vi "Redundant_Main_Micro_Comm.vi"(0 "GEA2 Reference In":refnum<k24>, 1 "GEA Inputs":T1 {"Destination" format="%.0x"; "Source" format="%.0x"}, 2 "Standalone?":bool, 11 "Error In":errorcluster, 12 "Repeat Count":i32=10) -> (4 "GEA2 Reference Out":refnum<k24>, 10 "Heart Beat Response":string[](array[string]), 15 "Error Out":errorcluster)   [LabVIEW 2016, in "2015 VA Washer.lvlib"]
doc: "This vi can be used to read ERD every 1 sec for user selected repeat counts."
uses:
  Projects/2015 VA Washer.lvlib
  C:/Automation/DLLs/PC Dot Net/GeaCommunication.dll
  Common/LabVIEW GEA2 Toolkit/LabVIEW_GEA2_Toolkit.lvlibp/type defs/Source_Destination.ctl
  Common/LabVIEW GEA2 Toolkit/LabVIEW_GEA2_Toolkit.lvlibp/type defs/ERD Read Data In.ctl
  Common/LabVIEW GEA2 Toolkit/LabVIEW_GEA2_Toolkit.lvlibp/type defs/Data Type.ctl
  Common/LabVIEW GEA2 Toolkit/LabVIEW_GEA2_Toolkit.lvlibp
panel:
  out "Pass/Fail":bool
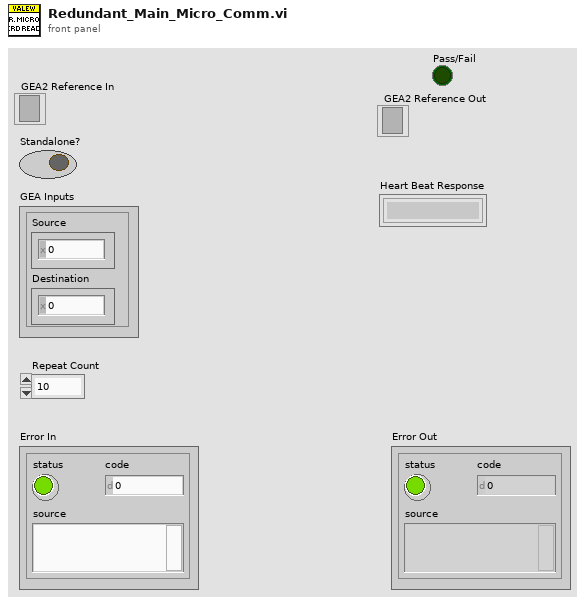
[diagram p1: front panel]
types:
  T1 = typedef "LabVIEW_GEA2_Toolkit.lvlibp/Source_Destination.ctl" = cluster{"Source":u8, "Destination":u8}
  T2 = typedef "LabVIEW_GEA2_Toolkit.lvlibp/ERD Read Data In.ctl" = cluster{"ERD Number":u16, "Data Type":T3}
  T3 = typedef "LabVIEW_GEA2_Toolkit.lvlibp/Data Type.ctl" = enum16{"string", "boolean", "uint8_t", "uint16_t", "uint32_t", "uint64_t", "int8_t", "int16_t", "int32_t", "int64_t"}
  T4 = typedef "LabVIEW_GEA2_Toolkit.lvlibp/ERD Read Data Out.ctl" = cluster{"ERD Number":u16, "Data":string}
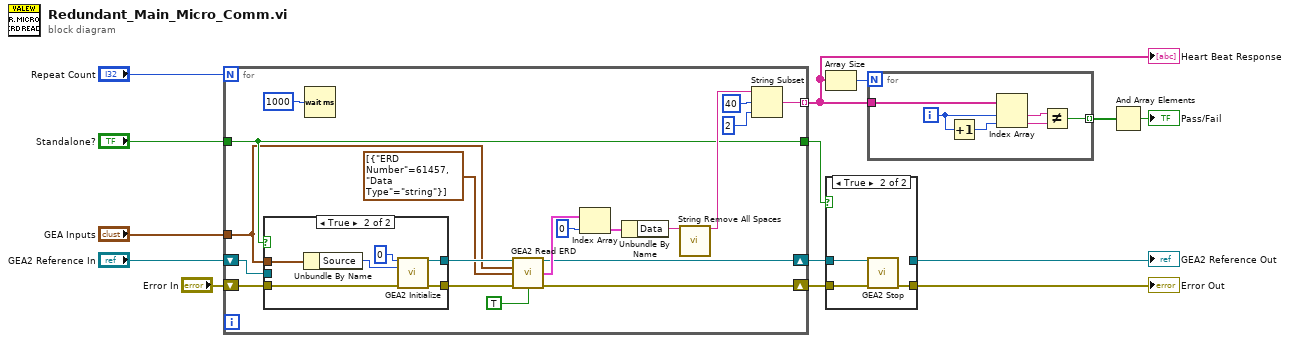
[diagram p0: block diagram]
diagram:
  n1 = for {
    N: "Repeat Count" -> [_]
    tunnel: [w24] -> w13
    tunnel: "Standalone?" -> [w24]
    tunnel: "GEA Inputs" -> [w19]
    shift-right: [w17] -> w10
    shift-left: "GEA2 Reference In" -> [w22]
    shift-right: [w16] -> w9
    shift-left: "Error In" -> [w21]
    tunnel: [w20] -> w3 mode=indexing
    n2 = case shown="True" w24 {
      tunnel: w21 -> [w34 w41]
      tunnel: [w34 w40] -> w33
      tunnel: w22 -> [w35 _]
      tunnel: [w35 w39] -> w32
      tunnel: w19 -> [_ w37]
      frame False {
      }
      frame True {
        n3 = Unbundle By Name(w37) -> ("Source"=w38:u8)
        n4 = call "GEA2 Initialize.vi"("Board Index"=0, "Source Address"=w38, "error in"=w41) -> ("GEA2 Reference Out"=w39:refnum<k24>, "error out"=w40:errorcluster)  [unwired: 10 in, 1 out]
      }
    }
    n5 = Wait (ms)(milliseconds to wait=u32 1000) -> ()  [unwired: 1 out]
    n6 = call "GEA2 Read ERD.vi"("GEA2 Reference In"=w32, "GEA Inputs"=w19, "Read ERD List"=T2[] [{"ERD Number"=61457, "Data Type"=enum."string"}], "Error In"=w33, "Verify ERD Response?"=TRUE) -> ("GEA2 Reference Out"=w17:refnum<k24>, "ERD Data Out"=w30:T4[], "Error Out"=w16:errorcluster)  [unwired: 7 in, 1 out]
    n7 = Index Array(array=w30, index=0) -> (element=w28:T4)
    n8 = Unbundle By Name(w28) -> ("Data"=w31:string)
    n9 = call "String Remove All Spaces.vi"("Input String"=w31) -> ("Spaces Removed"=w27:string)  [unwired: 13 in, 1 out]
    n10 = String Subset(string=w27, offset (0)=40, length (rest)=2 ("length (rest)")) -> (substring=w20:string)
  }
  "Heart Beat Response" <- w3
  n11 = Array Size(array=w3) -> (size(s)=w4:i32)
  n12 = case shown="True" w13 {
    tunnel: [w43 w46] -> w14
    tunnel: w10 -> [w42 w45]
    tunnel: w9 -> [w43 w44]
    tunnel: [w42 _] -> w6
    frame False {
    }
    frame True {
      n13 = call "GEA2 Stop.vi"("GEA2 Reference In"=w45, "Error In"=w44) -> ("Error Out"=w46:errorcluster)  [unwired: 13 in]
    }
  }
  "Error Out" <- w14
  "GEA2 Reference Out" <- w6
  n14 = for {
    N: w4 -> [_]
    tunnel: w3 -> [w52]
    tunnel: [w47] -> w2 mode=indexing
    i -> [w50]
    n15 = Increment(x=w50) -> (x+1=w49:i32)
    n16 = Index Array(array=w52, index #1=w50, index #2=w49) -> (element #1=w51:string, element #2=w48:string)
    n17 = Not Equal?(x=w51, y=w48) -> (x != y?=w47:bool)
  }
  n18 = And Array Elements(Boolean array=w2) -> (logical AND=→"Pass/Fail":bool)
